vi "Distance Drive Mode.vi"(0 "Y Output High":dbl, 1 "Y Output Low":dbl, 2 "X Output High":dbl, 3 "X Output Low":dbl, 5 "Y target":dbl, 9 "Heading target":dbl, 11 "Strafe target":dbl, 12 "Reinitialize":bool) -> (4 "isFinished":bool, 6 "Y out":dbl, 10 "Strafe out":dbl, 14 "Dist Drive Status":T1, 15 "X out":dbl)   [LabVIEW 2014]
uses:
  Common Code/Dist Drive Status.ctl
  Drivetrain Output Range.ctl
  Common Code/Change Detect Double.vi
  Robot Global Data.vi
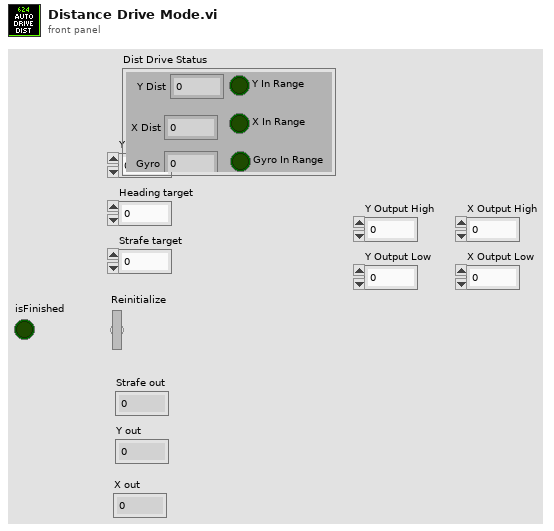
[diagram p1: front panel]
types:
  T1 = typedef "Dist Drive Status.ctl" = cluster{"Y In Range":bool, "X In Range":bool, "Gyro In Range":bool, "Y Dist":dbl, "X Dist":dbl, "Gyro":dbl}
  T2 = typedef "Drivetrain Output Range.ctl" = cluster{"output high":dbl, "output low":dbl}
  T3 = typedef "Dashboard Control Data.ctl" = cluster{"Cam Exposure":dbl, "Go to angle":dbl, "Steer PID Gains":cluster{"proportional gain (Kc)":dbl, "integral time (Ti, min)":dbl, "derivative time (Td, min)":dbl}, "Steer PID output Range":cluster{"output high":dbl, "output low":dbl}, "Pressure m \nValue":dbl, "Pressure b \nValue":dbl, "Roller Command Cluster ":T4, "Elevator":T5, "Encoder Control":T7, "Auton Settings":cluster{"Drive Dist Window Size":dbl}, "Drivetrain Settings":T8, "Lance":T9}
  T4 = typedef "Roller Control.ctl" = cluster{"Intake Speed":dbl, "Turn In Speed":dbl, "Unload Speed":dbl, "Turn Out Speed":dbl, "Ping Align Tolerance":dbl, "Tote Range Threshold":dbl, "Right Pot 0":dbl, "Pot Threshold":dbl, "Left Pot 0":dbl, "Manual 0s?":bool, "Right Pot Scale":dbl, "Left Pot Scale":dbl, "0 wait time":i32, "Zero Pots":bool, "Min Elevator Height":dbl, "Eject Time":dbl, "Eject US Threshold":dbl, "Anti-Twitch Time":u32, "Ping Caring Threshold":dbl, "Pot Diff Threshold":dbl, "Pinch Sustain":u32, "Absorb Give Up Threshold":dbl, "Untip In Threshold":dbl, "Untip Grab Range":dbl, "Ultrasonic Hold Time":u32, "Landscape Absorb Time":u32, "Pot Use Wait Time":u32, "Can Turn Stop Range":dbl, "Ignore Pressure":bool, "HP Load Speed":dbl}
  T5 = typedef "Elevator DB Control.ctl" = cluster{"PID Output Range":cluster{"output high":dbl, "output low":dbl}, "PID gains":cluster{"proportional gain (Kc)":dbl, "integral time (Ti, min)":dbl, "derivative time (Td, min)":dbl}, "Height Tolerance":sgl, " Encoder Constant":dbl, "Safe Mode Max Speed":sgl, "Eject Time":sgl, "Zeroing Speed":sgl, "Presets":T6, "Ping Detect Threshold":sgl, "Trashcan Detect Threshold":sgl, "Zero Filter Time":dbl, "Stabilizer Open Time":dbl, "Zero Creep Speed":dbl, "Max Current":dbl, "Current Trip Time":dbl, "Abort Pitch":dbl, "Finger m":dbl, "Finger b":dbl, "Finger max ":dbl, "Finger Stabilizer":dbl, "Finger Store":dbl, "Finger Stop Store":dbl, "Stabilizer Close Time":dbl, "HP Finger Store":dbl, "HP Finger Stop Store":dbl, "Finger min":dbl, "Unstick gain":dbl, "Roller Wait":dbl}
  T6 = typedef "Elevator Presets.ctl" = cluster{"Pickup 2 w/ Tote":sgl, "Pickup 2 w/ Trashcan":sgl, "Pickup 3 w/ Tote":sgl, "Pickup 3 w/ Trashcan":sgl, "Bottom":sgl, "Pickup 1 w/ Tote":sgl, "Pickup Trashcan":sgl, "Pickup 1 w/ Trashcan":sgl, "Eject":sgl, "Hold Low":sgl, "Step add height":sgl, "Untip Lift":dbl, "Drop Stack":dbl, "HP Load Hold":dbl, "HP Load Drop":dbl, "HP Load Finger":dbl, "HP Load Hold Can":dbl, "Store can max":dbl, "HP Drag Score":dbl, "HP Store can max":dbl, "HP Drag Finish":dbl, "HP Carry min":dbl, "HP Finger Anti-Crash":dbl, "Finger trashcan avoid":dbl}
  T7 = typedef "Encoder Control.ctl" = cluster{"Left Tick Constant":dbl, "Right Tick Constant":dbl, "Center Tick Constant":dbl, "Reset?":bool, "Y Dist":cluster{"PID gains":cluster{"proportional gain (Kc)":dbl, "integral time (Ti, min)":dbl, "derivative time (Td, min)":dbl}}, "X Dist":cluster{"PID gains":cluster{"proportional gain (Kc)":dbl, "integral time (Ti, min)":dbl, "derivative time (Td, min)":dbl}}, "Y Stop Thresh":dbl, "Y Stop Speed":dbl, "X Stop Thresh":dbl, "X Stop Speed":dbl}
  T8 = typedef "Drivetrain Settings.ctl" = cluster{"Gyro Tolerance":sgl, "Strafe Correct max steer":sgl, "Strafe Timer Wait":sgl, "Throttle Ramp (ms)":sgl, "Strafe Ramp (ms)":sgl, "Angular rate compensation":bool, "Throttle to Rate Scale":sgl, "Rate compensation gain":sgl, "Creep Steer":sgl, "Creep Throttle":sgl}
  T9 = typedef "Pike DB Controls.ctl" = cluster{"Down Speed":dbl, "Up Speed":dbl, "Max Down Time":dbl, "Max Up Time":dbl, "Current Limit":dbl}
  T10 = typedef "Encoder Values SuperCluster.ctl" = cluster{"Left Encoder":T11, "Center Encoder":T11, "Right Encoder":T11}
  T11 = typedef "Encoder Values.ctl" = cluster{"Distance":dbl, "Speed":dbl, "Ticks":dbl}
  T12 = cluster{"PID gains":cluster{"proportional gain (Kc)":dbl, "integral time (Ti, min)":dbl, "derivative time (Td, min)":dbl}}
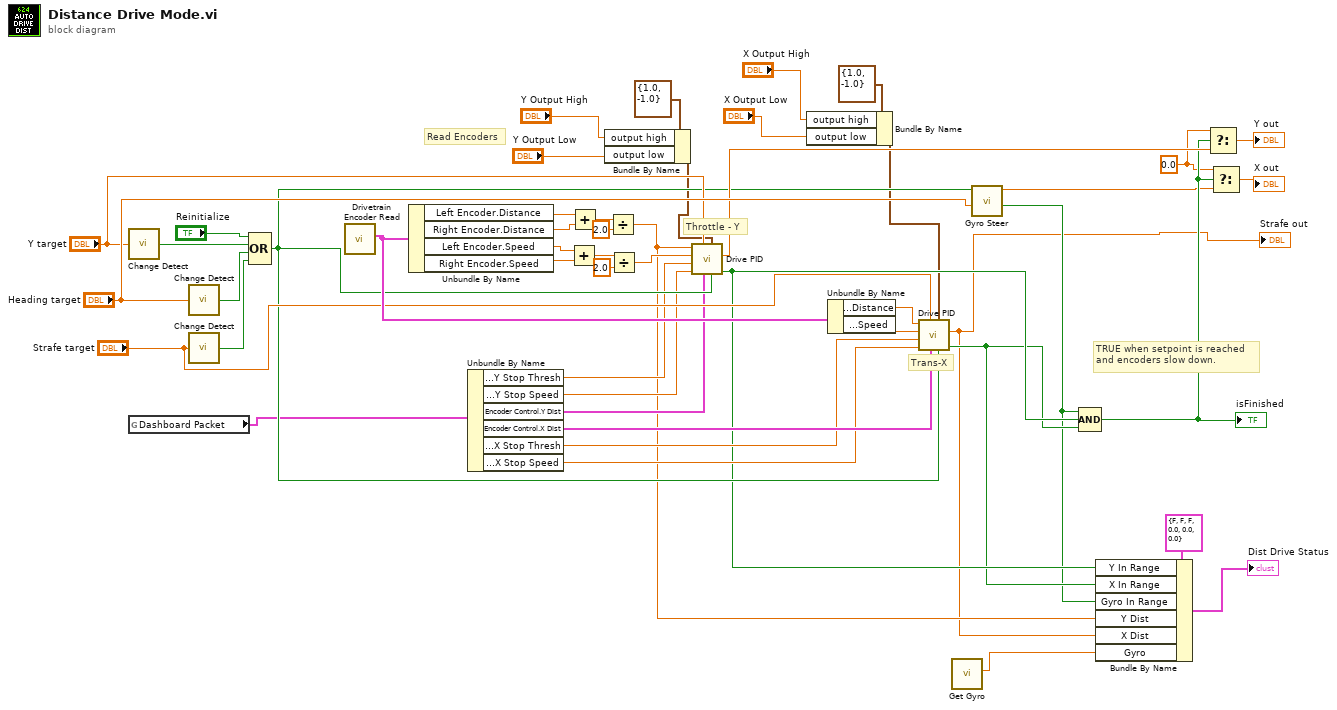
[diagram p0: block diagram]
diagram:
  w28 = 0.0 ("t")
  # "Throttle - Y"
  # "Trans-X"
  # "Read Encoders"
  # "TRUE when setpoint is reached\nand encoders slow down."
  n1 = call-poly "Change Detect.vi"("In"="Y target") -> ("Changed?"=w49:bool)
  n2 = global read "Robot Global Data.vi" "Dashboard Packet"() -> (w24:T3)
  n3 = call-poly "Change Detect.vi"("In"="Heading target") -> ("Changed?"=w48:bool)
  n4 = call-poly "Change Detect.vi"("In"="Strafe target") -> ("Changed?"=w47:bool)
  n5 = Compound Arithmetic op=OR("Reinitialize", w49, w48, w47) -> (w25:bool)
  n6 = call "Drivetrain Encoder Read.vi"() -> ("Quick use cluster"=w43:T10)  [unwired: 11 in]
  n7 = Unbundle By Name(w43) -> ("Left Encoder.Distance"=w38:dbl, "Right Encoder.Distance"=w39:dbl, "Left Encoder.Speed"=w41:dbl, "Right Encoder.Speed"=w40:dbl)
  n8 = Unbundle By Name(w24) -> ("Encoder Control.Y Stop Thresh"=w19:dbl, "Encoder Control.Y Stop Speed"=w18:dbl, "Encoder Control.Y Dist"=w23:T12, "Encoder Control.X Dist"=w22:T12, "Encoder Control.X Stop Thresh"=w21:dbl, "Encoder Control.X Stop Speed"=w20:dbl)
  n9 = Add(x=w41, y=w40) -> (x+y=w34:dbl)
  n10 = Add(x=w38, y=w39) -> (x+y=w37:dbl)
  n11 = Bundle By Name(cluster=T2 {"output high"=1.0, "output low"=-1.0} ("output range"), "output high"="Y Output High", "output low"="Y Output Low") -> (w3:T2)
  n12 = Divide(x=w37, y=2.0) -> (x/y=w12:dbl)
  n13 = Divide(x=w34, y=2.0) -> (x/y=w33:dbl)
  n14 = call "Drive PID.vi"("reinitialize? (F)"=w25, "output range"=w3, "PID Params"=w23, "Setpoint"="Y target", "Max Stop Speed"=w18, "Distance Stop Threshold"=w19, "Current Speed"=w33, "Current Distance"=w12) -> ("Finished"=w15:bool, "output"=w30:dbl)  [unwired: 2 in]
  n15 = Bundle By Name(cluster=T2 {"output high"=1.0, "output low"=-1.0} ("output range"), "output high"="X Output High", "output low"="X Output Low") -> (w2:T2)
  n16 = Unbundle By Name(w43) -> ("Center Encoder.Distance"=w26:dbl, "Center Encoder.Speed"=w27:dbl)
  n17 = call "Drive PID.vi"("reinitialize? (F)"=w25, "output range"=w2, "PID Params"=w22, "Setpoint"="Strafe target", "Max Stop Speed"=w20, "Distance Stop Threshold"=w21, "Current Speed"=w27, "Current Distance"=w26) -> ("Finished"=w14:bool, "output"=w11:dbl)  [unwired: 2 in]
  "Strafe out" <- w11
  n18 = call "Get Gyro.vi"() -> ("Angle"=w1:dbl)  [unwired: 11 in]
  n19 = call "Gyro Steer.vi"("Target Angle"="Heading target", "Changed?"=w25) -> ("In Range?"=w13:bool, "X out"=w10:dbl)  [unwired: 8 in]
  n20 = Compound Arithmetic op=AND(w13, w15, w14) -> (w29:bool)
  "isFinished" <- w29
  n21 = Bundle By Name(cluster=T1 {"Y In Range"=FALSE, "X In Range"=FALSE, "Gyro In Range"=FALSE, "Y Dist"=0.0, "X Dist"=0.0, "Gyro"=0.0} ("Dist Drive Status"), "Y In Range"=w15, "X In Range"=w14, "Gyro In Range"=w13, "Y Dist"=w12, "X Dist"=w11, "Gyro"=w1) -> (→"Dist Drive Status":T1)
  n22 = Select(t=w28, s=w29, f=w30) -> (s? t:f=→"Y out":dbl)
  n23 = Select(t=w28, s=w29, f=w10) -> (s? t:f=→"X out":dbl)
